vi "PH_Synchrolock_Watch.Set Default.vi"(0 "i ref in":refnum<vi>, 5 "error in":errorcluster) -> (14 "i ref out":refnum<vi>, 19 "error out":errorcluster)   [LabVIEW 2014, in "PH_Synchrolock_Watch.lvlib"]
doc: "This VI sets the hardware to default configuration."
uses:
  PH_Synchrolock_Watch.lvlib
  PH_TKTDS-30xx/PH_TKTDS-30xx.Channel Config.ctl
  PH_TKTDS-30xx/PH_TKTDS-30xx.Trigger Config.ctl
  PH_TKTDS-30xx/PH_TKTDS-30xx.Acquisition Config.ctl
  PH_TKTDS-30xx/PH_TKTDS-30xx.lvlib
panel:
  in  "Channel Settings":T2={"GUI Element Name"="", "Chan Settings"={"Channel Name"="CH1", "Input Impedance"="MEG", "Max Input Frequency"="TWENTY", "Vertical Coupling"=1, "Channel Enabled"=TRUE, "Probe Attenuation"=1.0, "Vertical Range"=100.0, "Vertical Offset"=0.0}} {"Chan Settings"."Vertical Offset" format="%#_6p"; "Chan Settings"."Vertical Range" items=["1mV"=0.001, "2mV"=0.002, "5mV"=0.005, "10mV"=0.01, "20mV"=0.02, "50mV"=0.05, "100mV"=0.1, "200mV"=0.2, "500mV"=0.5, "1V"=1.0]; "Chan Settings"."Probe Attenuation" format="%#.2f"}
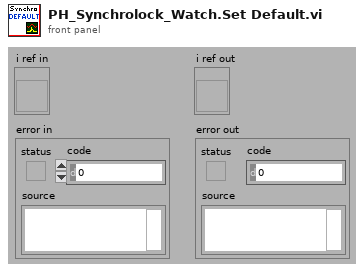
[diagram p1: front panel]
types:
  T1 = typedef "PH_TKTDS-30xx.lvlib/PH_TKTDS-30xx.Channel Config.ctl" = cluster{"Channel Name":string, "Input Impedance":string, "Max Input Frequency":string, "Vertical Coupling":i32, "Channel Enabled":bool, "Probe Attenuation":dbl, "Vertical Range":dbl, "Vertical Offset":dbl}
  T2 = cluster{"GUI Element Name":string, "Chan Settings":T1}
  T3 = typedef "PH_TKTDS-30xx.lvlib/PH_TKTDS-30xx.Acquisition Config.ctl" = cluster{"Time base":dbl, "Record Length":u16, "Start Time":dbl, "Type":i32, "Continuous":bool}
  T4 = typedef "PH_TKTDS-30xx.lvlib/PH_TKTDS-30xx.Trigger Config.ctl" = cluster{"Source":string, "Slope":i32, "Level [V]":dbl}
  T5 = typedef "PH_TKTDS-30xx.lvlib/PH_TKTDS-30xx.i attribute.ctl" = cluster{"Default VISA Resource":string, "VISA Resource Name":refnum<visa-resource-name>, "Revision":cluster{"Instrument Driver":string, "Instrument Firmware":string}, "Selftest":cluster{"Result":u32, "Message":string}, "Channels":T1[], "Trigger Configuration":T4, "Acquisition Configuration":T3, "Fetched Waveforms":T6[], "GUI Refs":T7, "GUI Refs Channels":refnum<vi>[], "State":T8, "Error Message":string, "Allow Prdc Loop?":bool}
  T6 = typedef "PH_TKTDS-30xx.lvlib/PH_TKTDS-30xx.fetched Waveform.ctl" = cluster{"Source":string, "Actual Points":u32, "Initial X":dbl, "X Increment":dbl, "Waveform Array":dbl[]}
  T7 = typedef "PH_TKTDS-30xx.lvlib/PH_TKTDS-30xx.GUI Refs.ctl" = cluster{"Trigger":refnum<vi>, "Acquisition":refnum<vi>, "Graph":refnum<vi>, "State":refnum<vi>, "Delete":refnum<vi>, "Channel to be positioned":refnum<vi>, "Postion":refnum<vi>, "Display Intensity":refnum<vi>, "VISA Resource":refnum<vi>}
  T8 = typedef "PH_StatusHandler.lvlib/PH_StatusHandler.Status.ctl" = i16
  T9 = cluster{"GUI Element Name":string, "Chan Settings":T1}[]
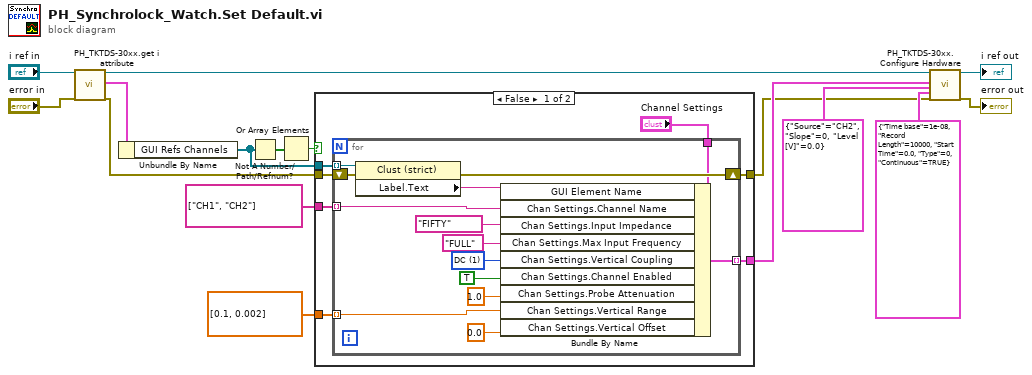
[diagram p0: block diagram]
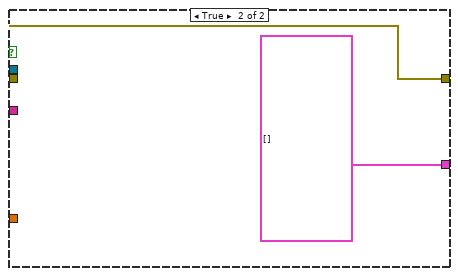
[diagram p2: hidden frame]
diagram:
  w5 = dbl[] [0.1, 0.002] items=["1mV"=0.001, "2mV"=0.002, "5mV"=0.005, "10mV"=0.01, "20mV"=0.02, "50mV"=0.05, "100mV"=0.1, "200mV"=0.2, "500mV"=0.5, "1V"=1.0]
  n1 = call "PH_TKTDS-30xx.get i attribute.vi"("i ref in"="i ref in", "error in (no error)"="error in") -> ("i ref out"=w10:refnum<vi>, "i attribute"=w9:T5, "error out"=w7:errorcluster)  [unwired: 15 in]
  n2 = Unbundle By Name(w9) -> ("GUI Refs Channels"=w3:refnum<vi>[])
  n3 = Not A Number/Path/Refnum?(number/path/refnum=w3) -> (NaN/Path/Refnum?=w2:bool[])
  n4 = Or Array Elements(Boolean array=w2) -> (logical OR=w1:bool)
  n5 = case shown="False" w1 {
    tunnel: [w23 T9 []] -> w8
    tunnel: w7 -> [w22 w38]
    tunnel: [w21 w38] -> w6
    tunnel: w5 -> [w20 _]
    tunnel: string[] ["CH1", "CH2"] -> [w19 _]
    tunnel: w3 -> [w18 _]
    frame False {
      n6 = for {
        tunnel: w18 -> [w37] mode=indexing
        shift-right: [w35] -> w21
        shift-left: w22 -> [w36]
        tunnel: "Channel Settings" -> [w33]
        tunnel: [w34] -> w23 mode=indexing
        tunnel: w20 -> [w32] mode=indexing
        tunnel: w19 -> [w31] mode=indexing
        w24 = 1 items=["AC", "DC", "GND"] ("Vertical Coupling")
        n7 = property class="Clust (strict)"(reference=w37, error in=w36) -> (error out=w35:errorcluster, "Label.Text"=w30:string)  [unwired: 1 out]
        n8 = Bundle By Name(cluster=w33, "GUI Element Name"=w30, "Chan Settings.Channel Name"=w31, "Chan Settings.Input Impedance"="FIFTY" ("Input Impedance"), "Chan Settings.Max Input Frequency"="FULL" ("Max Input Frequency"), "Chan Settings.Vertical Coupling"=w24, "Chan Settings.Channel Enabled"=TRUE, "Chan Settings.Probe Attenuation"=1.0, "Chan Settings.Vertical Range"=w32, "Chan Settings.Vertical Offset"=0.0) -> (w34:T2)
      }
    }
    frame True {
    }
  }
  n9 = call "PH_TKTDS-30xx.Configure Hardware.vi"("i ref in"=w10, "Channels Sets"=w8, "Trigger Settings"=T4 {"Source"="CH2", "Slope"=0, "Level [V]"=0.0}, "Acqu Settings"=T3 {"Time base"=1e-08, "Record Length"=10000, "Start Time"=0.0, "Type"=0, "Continuous"=TRUE}, "error in"=w6) -> ("i ref out"=→"i ref out":refnum<vi>, "error out"=→"error out":errorcluster)  [unwired: 13 in]
